vi "ds get firmware version.vi"(10 "dest":cluster{}, 11 "device_handle":u32) -> (1 "function return":i32, 2 "dest out":cluster{}, 3 "device_handle out":u32)   [LabVIEW 2019, in "apdm.lvlib"]
doc: "APDM_EXPORT int apdm_ds_get_firmware_version(apdm_device_handle_t device_handle, uint64_t *dest);"
uses:
  apdm.lvlib
  Lee Lab/CP FES Walking 2018/Code/Working/LabVIEW/apdm.dll
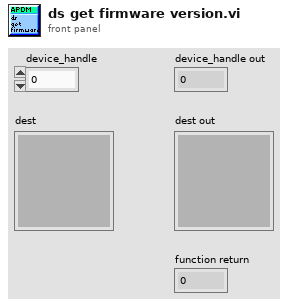
[diagram p1: front panel]
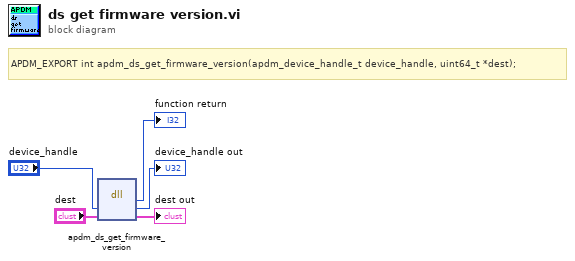
[diagram p0: block diagram]
diagram:
  # "APDM_EXPORT int apdm_ds_get_firmware_version(apdm_device_handle_t device_handle, uint64_t *dest);"
  n1 = dll-call lib="C:/Users/jfalesi/Dropbox/Lee Lab/CP FES Walking 2018/Code/Working/LabVIEW/apdm.*" fn="apdm_ds_get_firmware_version"("device_handle"="device_handle", "dest"="dest") -> (→"function return":i32, "device_handle"=→"device_handle out":u32, "dest"=→"dest out":cluster{})  [unwired: 3 in, 2 out]
